vi "testQue.vi"   [LabVIEW 2009, in "run.lvlib"]
uses:
  run.lvlib
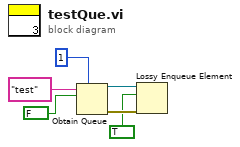
[diagram p0: block diagram]
diagram:
  n1 = Obtain Queue(max queue size (-1, unlimited)=1, name (unnamed)="test", element data type=FALSE) -> (queue out=w2:refnum<queue>, error out=w3:errorcluster)  [unwired: 2 in, 1 out]
  n2 = Lossy Enqueue Element(queue=w2, element=TRUE, error in (no error)=w3) -> ()  [unwired: 4 out]
